vi "Do.vi"(8 "error in (no error)":errorcluster, 10 "Actor in":refnum<class "Actor.lvclass">, 11 "ControlHumidifierPump":refnum<class "ControlHumidifierPump.lvclass">) -> (0 "error out":errorcluster, 2 "Actor out":refnum<class "Actor.lvclass">)   [LabVIEW 2014, in "Controller.lvlib" / "ControlHumidifierPump.lvclass"]
doc: "(<B>Filename</B>: Actor Framework.lvlib:Message.lvclass:Do.vi)\n\nDefines what a message does when it is received by an actor. Generally, a message instructs an actor to invoke one of its methods. By default, this method does nothing. A child class must override it to define behavior. Create a child class by using the Actor Framework Message Maker dialog box."
uses:
  ControlHumidifierPump.lvclass
  <vilib>/ActorFramework/Actor/Actor.lvclass
  ControlHumidifierPump.lvclass/ControlHumidifierPump.ctl
  Controller.lvclass
  SuperActor/SuperActor.lvclass/SuperActor.ctl
  <vilib>/DAQmx/write.llb/DAQmx Write (Digital Bool 1Line 1Point).vi
  SuperActor/Read Log Session.vi
  <vilib>/DAQmx/miscellaneous.llb/DAQmx Fill In Error Info.vi
  <userlib>/_Session Fwk/Session - Root.lvclass
  reusable/Session APIs/Session Log/System Log.lvclass
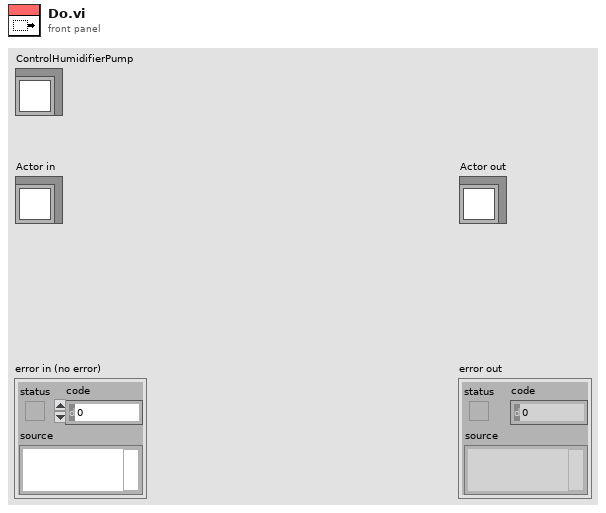
[diagram p1: front panel]
types:
  T1 = typedef "Session - Root.lvclass/Session Handle.ctl" = refnum<data-value>
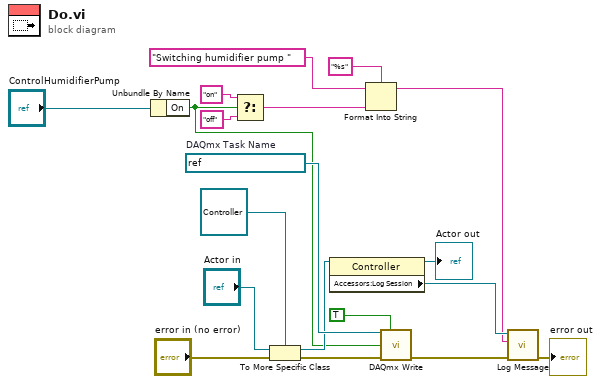
[diagram p0: block diagram]
diagram:
  w19 = refnum<k21> "Humidifier Pump"  # DAQmx Task Name
  n1 = Unbundle By Name("ControlHumidifierPump") -> ("On"=w1:bool)
  n2 = Select(t="on", s=w1, f="off") -> (s? t:f=w6:string)
  n3 = To More Specific Class(target class=refnum<class "Controller.lvclass"> refnum ("Controller.lvlib:Controller"), reference="Actor in", error in="error in (no error)") -> (specific class reference=w14:refnum<class "Controller.lvclass">, error out=w8:errorcluster)
  n4 = property class="Controller"(reference=w14) -> (reference out=→"Actor out":refnum<class "Controller.lvclass">, "Accessors:Log Session"=w13:T1)  [unwired: 1 in, 1 out]
  n5 = Format Into String(format string="%s", initial string="Switching humidifier pump " ("MSG In"), w6) -> (resulting string=w2:string)  [unwired: 1 in, 1 out]
  n6 = call-poly <vilib>:"DAQmx Write.vi"("task/channels in"=w19, "auto start"=TRUE, "data"=w1, "error in"=w8) -> ("error out"=w11:errorcluster)  [unwired: 9 in, 2 out]
  n7 = call "Log Message.vi"("error in"=w11, "MSG In"=w2, "session in"=w13) -> ("error out"=→"error out":errorcluster)  [unwired: 7 in, 1 out]
